vi "Get Self Cal.vi"(2 "shared":refnum<class "niUSRP Rx Core v1 FPGA.lvclass">=refnum) -> (4 "self cal":refnum<class "Self Cal.lvclass">)   [LabVIEW 2023]
doc: "this VI is an accessor for Timing Information that contains the shared resource for Time-Keeping used by Alginment."
uses:
  <instrlib>/niUSRP/Reference FPGA/Rx Core/niUSRP Rx Core v1 FPGA.lvclass
  <instrlib>/niVST/Self Cal/v2/FPGA/Self Cal.lvclass
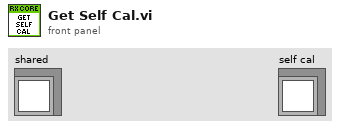
[diagram p1: front panel]
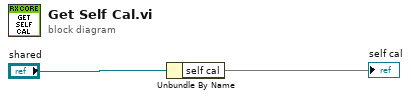
[diagram p0: block diagram]
diagram:
  n1 = Unbundle By Name("shared") -> ("self cal"=→"self cal")
